vi "Take Measurement.vi"(8 "error in (no error)":errorcluster, 10 "Transport in":refnum<class "Transport.lvclass">, 11 "SweepControl in":refnum<class "SweepControl.lvclass">) -> (0 "error out":errorcluster)   [LabVIEW 2016, in "SweepControl.lvclass"]
uses:
  SweepControl.lvclass
  Transport/Transport.lvclass
  SweepControl.lvclass/SweepControl.ctl
  Transport/Transport.lvclass/Transport.ctl
  Read Control Experiment.vi
  Control Experiment/Control Experiment.lvclass
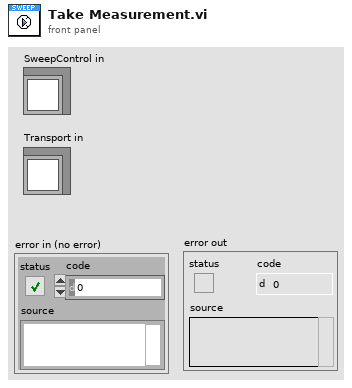
[diagram p1: front panel]
types:
  T1 = typedef "SweepControl.lvclass/Enum - Experiments.ctl" = enum16{"IV", "Lockin_time", "Lockin_Vsg", "Lockin (experimental)"}
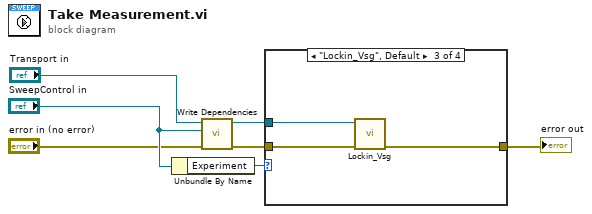
[diagram p0: block diagram]
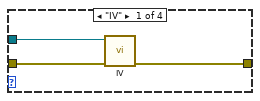
[diagram p2: hidden frame]
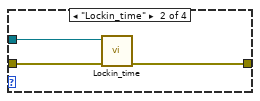
[diagram p3: hidden frame]
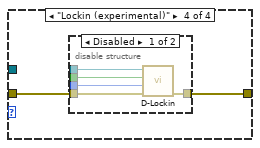
[diagram p4: hidden frame]
diagram:
  n1 = Unbundle By Name("SweepControl in") -> ("Experiment"=w3:T1)
  n2 = call "Write Dependencies.vi"("error in (no error)"="error in (no error)", "SweepControl"="SweepControl in", "Transport in"="Transport in") -> ("error out"=w6:errorcluster, "Transport out"=w4:refnum<class "Transport.lvclass">)  [unwired: 7 in]
  n3 = case shown="\"Lockin_Vsg\", Default" w3 {
    tunnel: w6 -> [w10 w13 w16 w18]
    tunnel: w4 -> [w9 w12 w15 _]
    tunnel: [w8 w11 w14 w17] -> w2
    frame "IV" {
      n4 = call "IV.vi"("error in"=w10, "Transport"=w9) -> ("error out"=w8:errorcluster)  [unwired: 8 in, 1 out]
    }
    frame "Lockin_time" {
      n5 = call "Lockin_time.vi"("error in (no error)"=w13, "Transport"=w12) -> ("error out"=w11:errorcluster)  [unwired: 8 in, 1 out]
    }
    frame "Lockin_Vsg", Default {
      n6 = call "Lockin_Vsg.vi"("error in (no error)"=w16, "Transport"=w15) -> ("error out"=w14:errorcluster)  [unwired: 8 in, 1 out]
    }
    frame "Lockin (experimental)" {
      n7 = disable-structure shown="Disabled" {
        disable-tunnel: _ -> [w23 _]
        disable-tunnel: w18 -> [w22 _]
        disable-tunnel: _ -> [w21 _]
        disable-tunnel: _ -> [w20 _]
        disable-tunnel: [w19 _] -> w17
        frame Disabled {
          n8 = call "D-Lockin.vi"("error in (no error)"=w22, "index"=w21, "Stop?"=w20, "SweepControl"=w23) -> ("error out"=w19:errorcluster)  [unwired: 6 in, 1 out]
        }
        frame Enabled {
        }
      }
    }
  }
  "error out" <- w2
